vi "Pre Launch Init.vi"(11 "IED Status Logger in":refnum<class "IED Status Logger.lvclass">) -> (0 "error out":errorcluster, 3 "IED Status Logger out":refnum<class "IED Status Logger.lvclass">)   [LabVIEW 2018, in "IED Status Logger Actor.lvlib" / "IED Status Logger.lvclass"]
doc: "(<B>Filename</B>: Actor Framework.lvlib:Actor.lvclass:Pre Launch Init.vi)\n\nDefines behavior that occurs after the Launch Nested Actor method is invoked but before the actor's Actor Core method begins running.\n\nBy default, this method does nothing. A descendant class may override it to define behavior."
uses:
  IED Status Logger.lvclass
  IED Status Logger.lvclass/IED Status Logger.ctl
  <vilib>/ActorFramework/Actor/Actor.lvclass
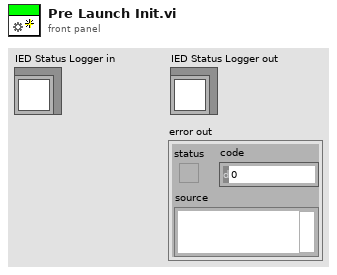
[diagram p1: front panel]
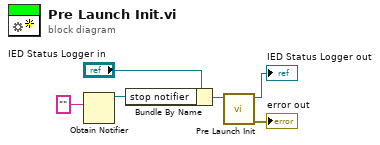
[diagram p0: block diagram]
diagram:
  n1 = Obtain Notifier(notification data type="") -> (notifier out=w1:refnum<notifier>)  [unwired: 3 in, 2 out]
  n2 = Bundle By Name(cluster="IED Status Logger in", "stop notifier"=w1) -> (w2:refnum<class "IED Status Logger.lvclass">)
  n3 = call-parent "Pre Launch Init.vi"("Actor in"=w2) -> ("error out"=→"error out":errorcluster, "Actor out"=→"IED Status Logger out":refnum<class "IED Status Logger.lvclass">)  [unwired: 9 in]
